vi "Test Set Subpanels-- SMO Array -- Not Created.vi"(8 "error in":errorcluster) -> (0 "error out":errorcluster)   [LabVIEW 2019]
uses:
  <vilib>/addons/_JKI Toolkits/Caraya/classes/Test/Test.lvclass
  Maui 2.0/Maui 2.0.lvclass
  <vilib>/JKI/JKI SMO/SMO/SMO.lvclass
  C:/Program Files (x86)/National Instruments/LabVIEW 2020/vi.lib/JKI/JKI SMO/SMO/SMO.lvclass
  <vilib>/addons/_JKI Toolkits/Caraya/classes/Assert/Assert.lvclass
  <vilib>/JKI/JKI SMO/SMO/Typedefs/SMOState --Enum.ctl
  <vilib>/addons/_JKI Toolkits/Caraya/classes/Assert/Assert True.vi
  <vilib>/addons/_JKI Toolkits/Caraya/classes/Assert/Assert Equal Value_Variant.vi
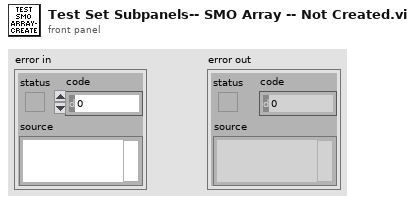
[diagram p1: front panel]
types:
  T1 = typedef "SMO.lvclass/SMOState --Enum.ctl" = enum16{"unknown", "Created", "Started", "Stopped"}
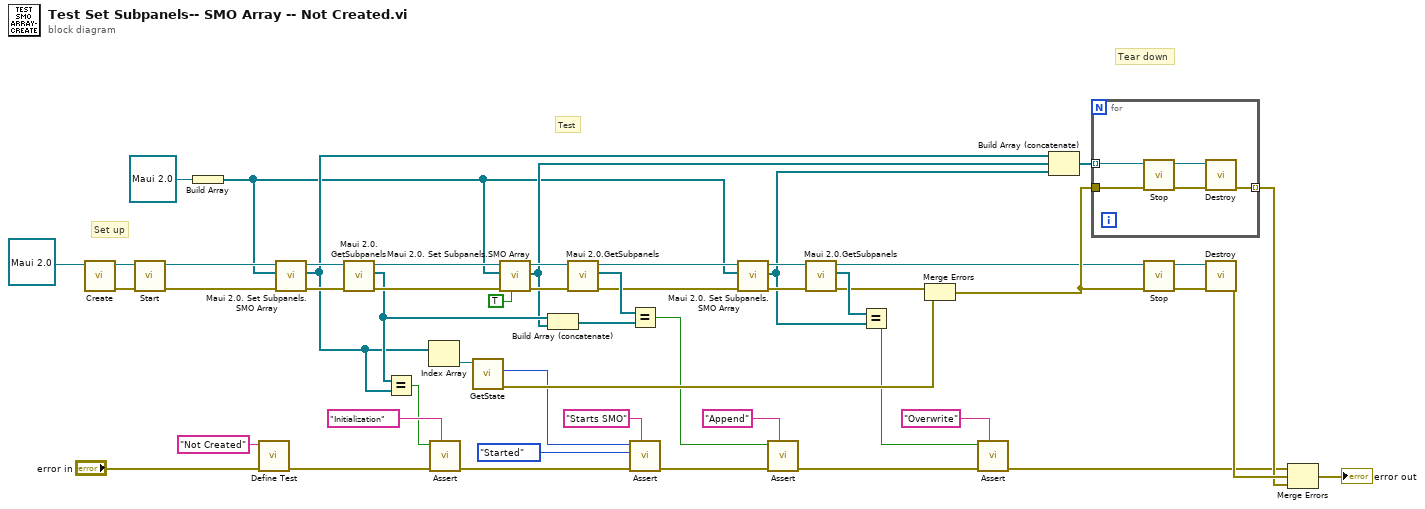
[diagram p0: block diagram]
diagram:
  # "Tear down"
  # "Test"
  # "Set up"
  n1 = call <vilib>:"Create.vi"("SMO"=refnum<class "Maui 2.0.lvclass"> refnum ("Maui 2.0.lvclass")) -> ("error out"=w48:errorcluster, "SMO out"=w47:refnum<class "Maui 2.0.lvclass">)  [unwired: 8 in, 1 out]
  n2 = call <vilib>:"Start.vi"("error in (no error)"=w48, "SMO"=w47) -> ("error out"=w45:errorcluster, "SMO out"=w44:refnum<class "Maui 2.0.lvclass">)  [unwired: 8 in]
  n3 = Build Array(refnum<class "Maui 2.0.lvclass"> refnum ("Maui 2.0.lvclass")) -> (w1:refnum<class "Maui 2.0.lvclass">[])
  n4 = call <vilib>:"Define Test.vi"("error in (no error)"="error in", "Label (VI Title)"="Not Created") -> ("error out"=w51:errorcluster)  [unwired: 9 in]
  n5 = call-dynamic "Maui 2.0. Set Subpanels.SMO Array.vi"("error in (no error)"=w45, "Subpanels in"=w1, "Maui 2.0 in"=w44) -> ("error out"=w36:errorcluster, "Subpanels Out"=w20:refnum<class "SMO.lvclass">[], "Maui 2.0 out"=w37:refnum<class "Maui 2.0.lvclass">)  [unwired: 6 in]
  n6 = call "Maui 2.0.GetSubpanels.vi"("error in (no error)"=w36, "Maui 2.0"=w37) -> ("error out"=w22:errorcluster, "Subpanels"=w21:refnum<class "SMO.lvclass">[], "Maui 2.0 out"=w23:refnum<class "Maui 2.0.lvclass">)  [unwired: 7 in]
  n7 = Equal?(x=w21, y=w20) -> (x = y?=w19:bool)
  n8 = Index Array(array=w20) -> (element=w34:refnum<class "SMO.lvclass">)  [unwired: 1 in]
  n9 = call-poly <vilib>:"Assert.vi"("Label"="Initialization", "error in (no error)"=w51, "True?"=w19) -> ("error out"=w31:errorcluster)  [unwired: 8 in]
  n10 = call <vilib>:"GetState.vi"("SMO"=w34) -> ("error out"=w30:errorcluster, "SMO State"=w3:T1)  [unwired: 8 in, 1 out]
  n11 = call-dynamic "Maui 2.0. Set Subpanels.SMO Array.vi"("Append (F)"=TRUE, "error in (no error)"=w22, "Subpanels in"=w1, "Maui 2.0 in"=w23) -> ("error out"=w25:errorcluster, "Subpanels Out"=w15:refnum<class "SMO.lvclass">[], "Maui 2.0 out"=w24:refnum<class "Maui 2.0.lvclass">)  [unwired: 5 in]
  n12 = Build Array (concatenate)(w21, w15) -> (w17:refnum<class "SMO.lvclass">[])
  n13 = call "Maui 2.0.GetSubpanels.vi"("error in (no error)"=w25, "Maui 2.0"=w24) -> ("error out"=w11:errorcluster, "Subpanels"=w18:refnum<class "SMO.lvclass">[], "Maui 2.0 out"=w8:refnum<class "Maui 2.0.lvclass">)  [unwired: 7 in]
  n14 = Equal?(x=w18, y=w17) -> (x = y?=w2:bool)
  n15 = call-poly <vilib>:"Assert.vi"("Label"="Starts SMO", "error in (no error)"=w31, "Y"=SMOState_--Enum."Started" ("SMO State"), "X"=w3) -> ("error out"=w33:errorcluster)  [unwired: 7 in]
  n16 = call-dynamic "Maui 2.0. Set Subpanels.SMO Array.vi"("error in (no error)"=w11, "Subpanels in"=w1, "Maui 2.0 in"=w8) -> ("error out"=w12:errorcluster, "Subpanels Out"=w4:refnum<class "SMO.lvclass">[], "Maui 2.0 out"=w13:refnum<class "Maui 2.0.lvclass">)  [unwired: 6 in]
  n17 = call-poly <vilib>:"Assert.vi"("Label"="Append", "error in (no error)"=w33, "True?"=w2) -> ("error out"=w27:errorcluster)  [unwired: 8 in]
  n18 = call "Maui 2.0.GetSubpanels.vi"("error in (no error)"=w12, "Maui 2.0"=w13) -> ("error out"=w9:errorcluster, "Subpanels"=w10:refnum<class "SMO.lvclass">[], "Maui 2.0 out"=w7:refnum<class "Maui 2.0.lvclass">)  [unwired: 7 in]
  n19 = Equal?(x=w10, y=w4) -> (x = y?=w6:bool)
  n20 = Merge Errors(w9, w30) -> (w29:errorcluster)
  n21 = call-poly <vilib>:"Assert.vi"("Label"="Overwrite", "error in (no error)"=w27, "True?"=w6) -> ("error out"=w26:errorcluster)  [unwired: 8 in]
  n22 = Build Array (concatenate)(w20, w15, w4) -> (w39:refnum<class "SMO.lvclass">[])
  n23 = for {
    tunnel: w39 -> [w55] mode=indexing
    tunnel: w29 -> [w54]
    tunnel: [w53] -> w38 mode=indexing
    n24 = call <vilib>:"Stop.vi"("error in (no error)"=w54, "SMO"=w55) -> ("error out"=w56:errorcluster, "SMO out"=w57:refnum<class "SMO.lvclass">)  [unwired: 8 in]
    n25 = call <vilib>:"Destroy.vi"("error in (no error)"=w56, "SMO"=w57) -> ("error out"=w53:errorcluster)  [unwired: 9 in]
  }
  n26 = call <vilib>:"Stop.vi"("error in (no error)"=w29, "SMO"=w7) -> ("error out"=w42:errorcluster, "SMO out"=w41:refnum<class "Maui 2.0.lvclass">)  [unwired: 8 in]
  n27 = call <vilib>:"Destroy.vi"("error in (no error)"=w42, "SMO"=w41) -> ("error out"=w40:errorcluster)  [unwired: 9 in]
  n28 = Merge Errors(w26, w40, w38) -> (→"error out":errorcluster)
